vi "arduinoDetachBasedOnTime.vi"(0 "delay (ms)":u32) -> ()   [LabVIEW 2012]
uses:
  GlobalArduino.vi
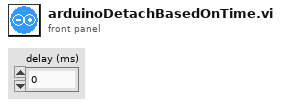
[diagram p1: front panel]
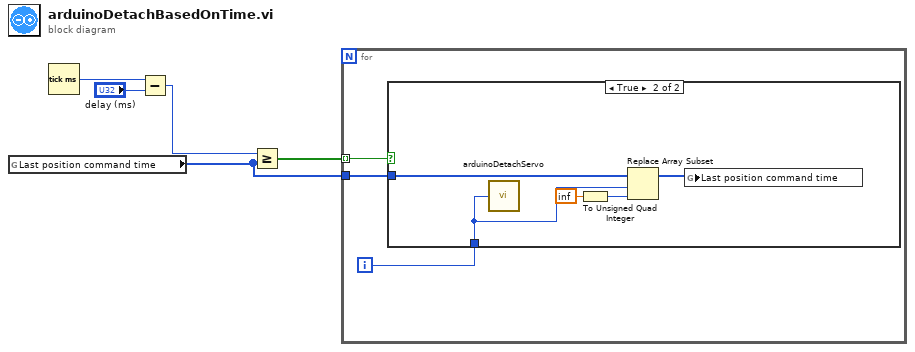
[diagram p0: block diagram]
diagram:
  n1 = global read "GlobalArduino.vi" "Last position command time"() -> (w1:u64[])
  n2 = Tick Count (ms)() -> (millisecond timer value=w5:u32)
  n3 = Subtract(x=w5, y="delay (ms)") -> (x-y=w3:u32)
  n4 = Greater Or Equal?(x=w3, y=w1) -> (x >= y?=w2:bool[])
  n5 = for {
    tunnel: w2 -> [w8] mode=indexing
    tunnel: w1 -> [w6]
    i -> [w7]
    n6 = case shown="True" w8 {
      tunnel: w7 -> [_ w11]
      tunnel: w6 -> [_ w12]
      frame False {
      }
      frame True {
        n7 = call "arduinoDetachServo.vi"("channel"=w11) -> ()
        n8 = To Unsigned Quad Integer(1:inf) -> (0:w9:u64)
        n9 = Replace Array Subset(array=w12, new element=w9, index=w11) -> (w13:u64[])
        n10 = global write "GlobalArduino.vi" "Last position command time"(w13) -> ()
      }
    }
  }
